vi "GetVehicleOrder.vi"(0 "Input String":string) -> (2 "Lane Offset":dbl, 3 "X":dbl, 4 "Y":dbl, 5 "Yaw":dbl, 14 "Vehicle Id":i32, 15 "Lane String":string, 16 "Is Cruise Control":bool, 17 "Velocity Value":dbl format="%#_13g", 18 "Desired Distance":dbl, 19 "Current Distance":dbl)   [LabVIEW 2013]
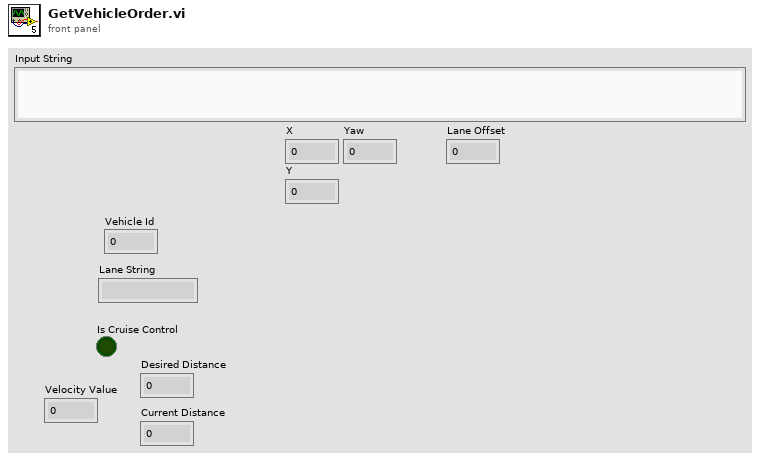
[diagram p1: front panel]
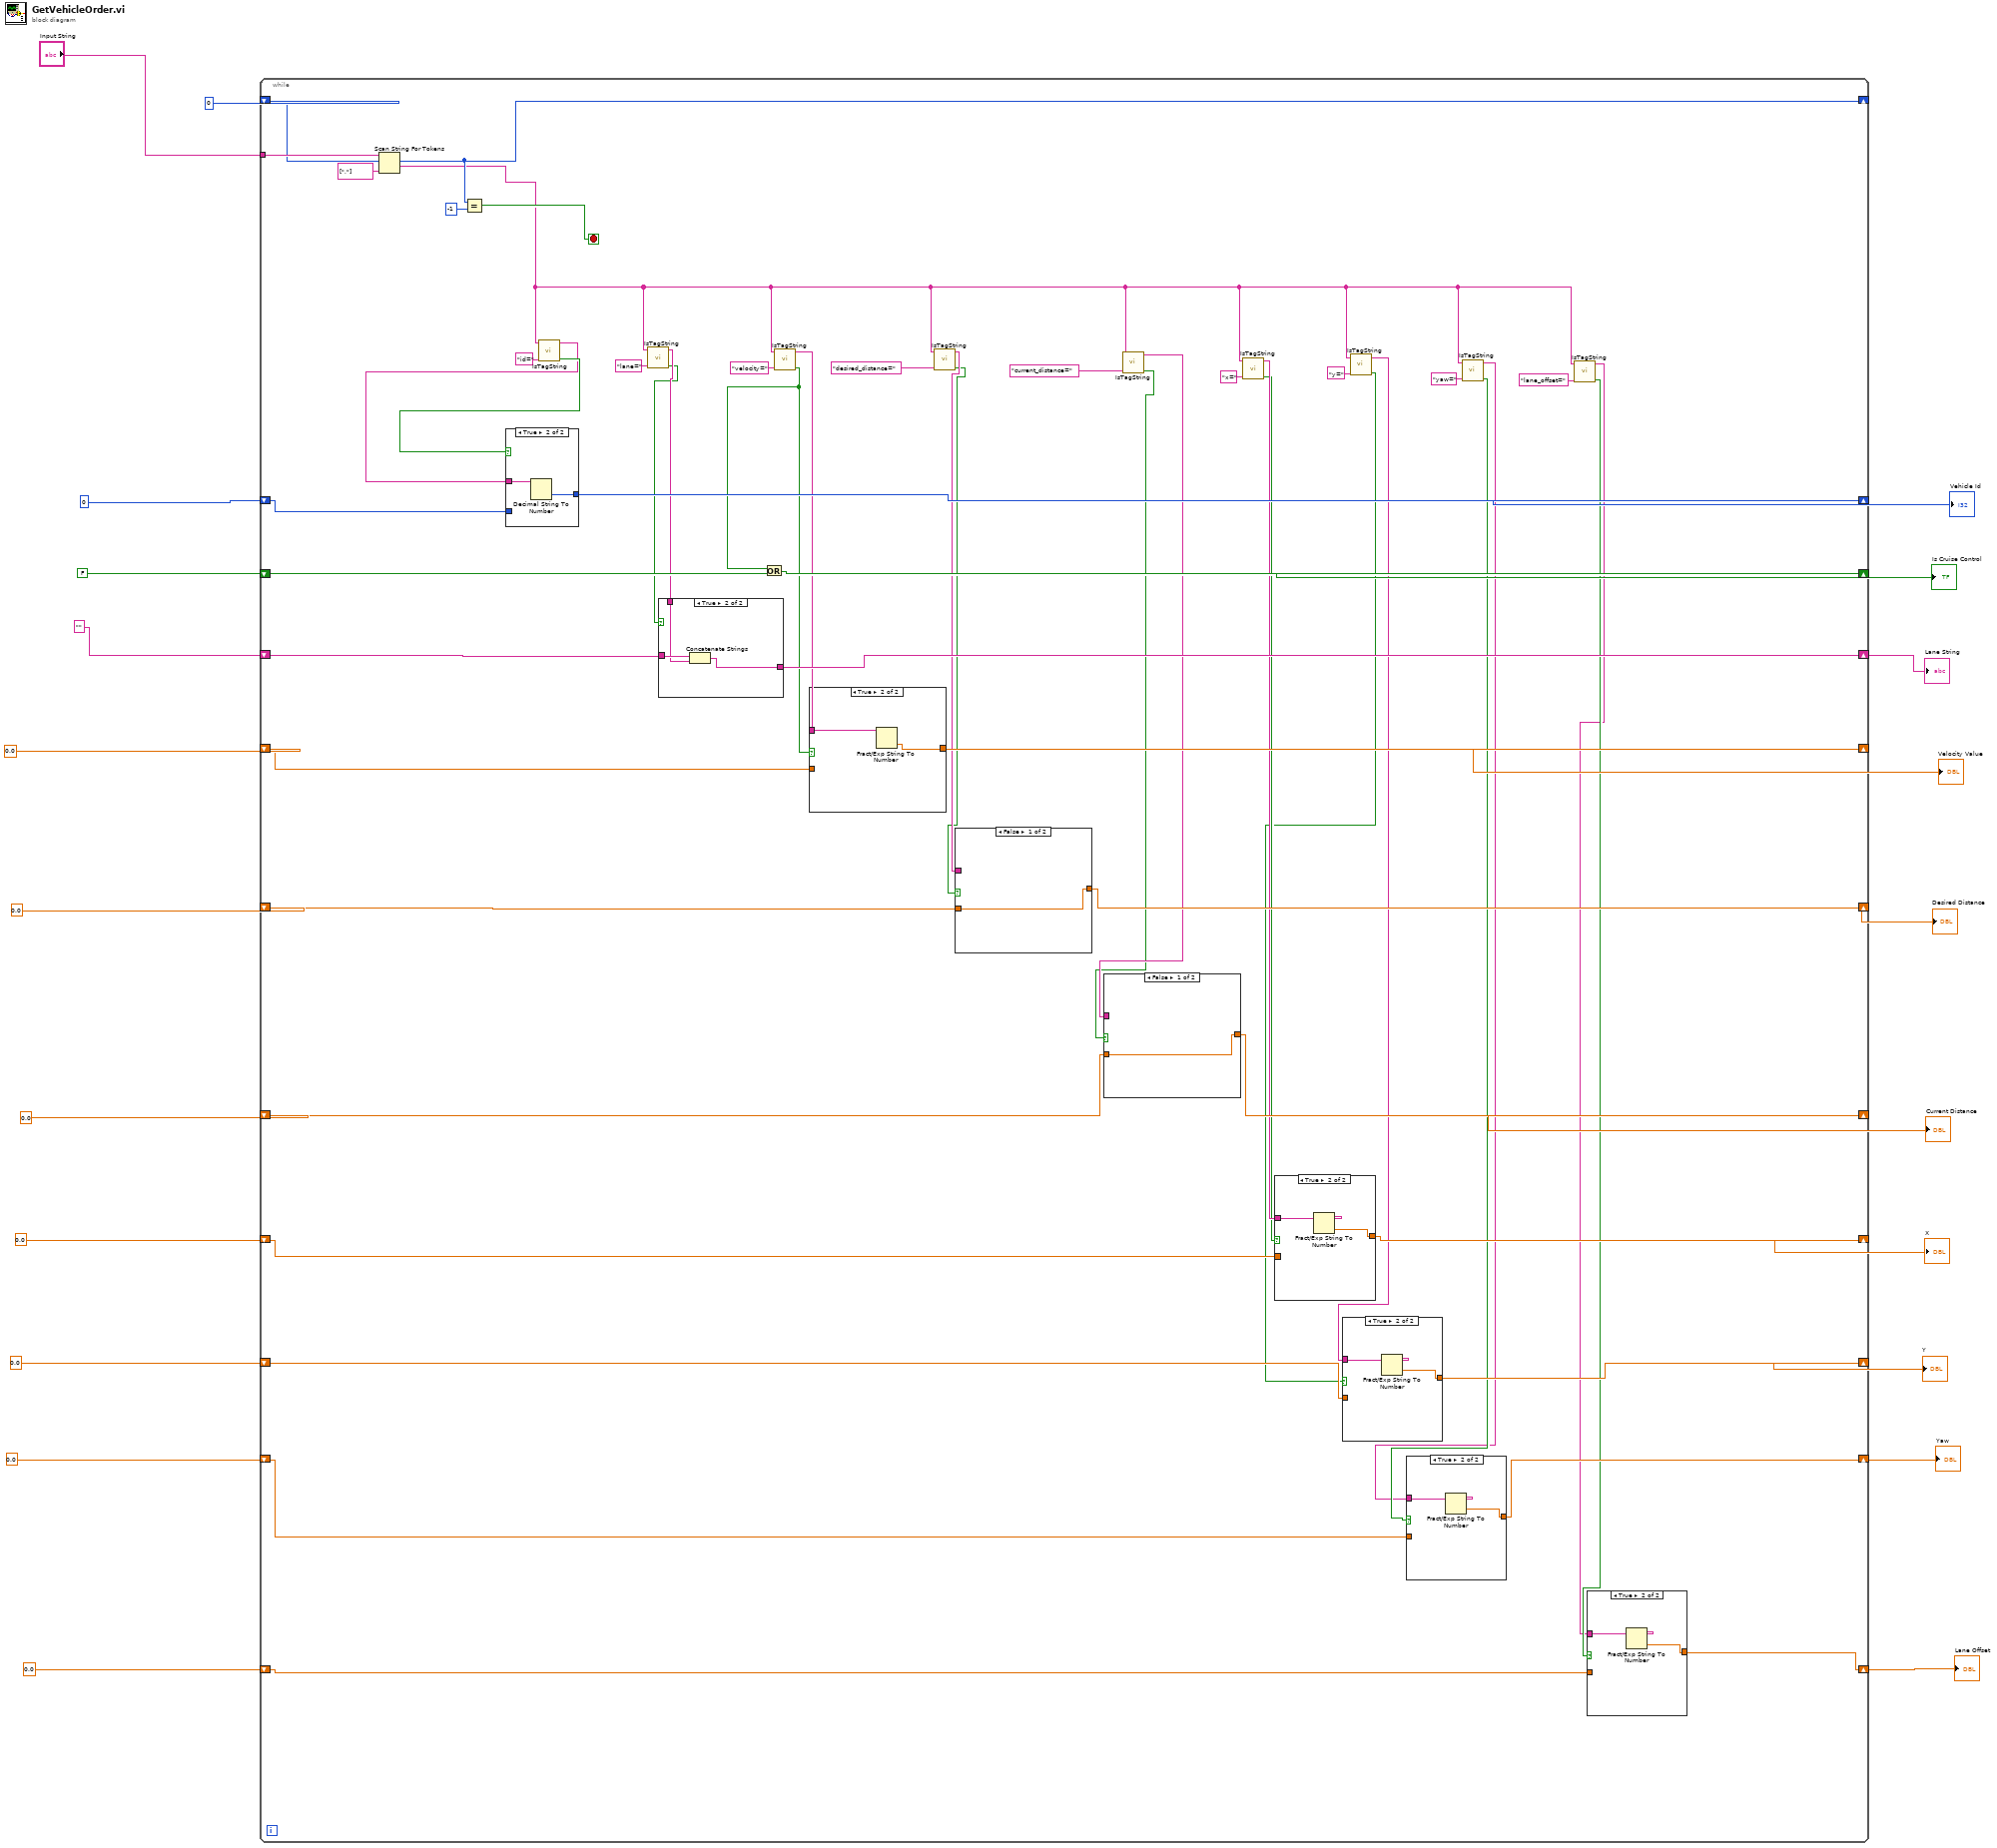
[diagram p0: block diagram]
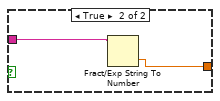
[diagram p6: hidden frame]
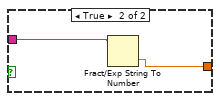
[diagram p7: hidden frame]
diagram:
  n1 = while {
    tunnel: "Input String" -> [w76]
    shift-right: [w49] -> _
    shift-left: 0 -> [w73]
    shift-right: [w66] -> w19
    shift-left: 0 -> [w65]
    shift-right: [w63] -> w17
    shift-left: FALSE -> [w64]
    shift-right: [w60] -> w16
    shift-left: "" -> [w61]
    shift-right: [w58] -> w14
    shift-left: 0.0 -> [w57]
    shift-right: [w55] -> w11
    shift-left: 0.0 -> [w56]
    shift-right: [w54] -> w10
    shift-left: 0.0 -> [w46]
    shift-right: [w37] -> w5
    shift-left: 0.0 -> [w38]
    shift-right: [w36] -> w4
    shift-left: 0.0 -> [w35]
    shift-right: [w33] -> w3
    shift-left: 0.0 -> [w34]
    shift-right: [w28] -> w1
    shift-left: 0.0 -> [w27]
    stop <- w74 stop-if-true
    n2 = Scan String For Tokens(6:string[] [","] ("delimiters (\\s,\\t,\\r,\\n)"), 8:w73, 9:w76) -> (1:w25:string, 2:w49:i32)  [unwired: 3 in, 2 out]
    n3 = Equal?(x=w49, y=-1) -> (x = y?=w74:bool)
    n4 = call "IsTagString.vi"("Input String"=w25, "Tag Desired"="id=") -> ("Value String"=w67:string, "Is Tag String"=w68:bool)  [unwired: 7 in]
    n5 = case shown="True" w68 {
      tunnel: w67 -> [_ w104]
      tunnel: [w102 w103] -> w66
      tunnel: w65 -> [w102 _]
      frame False {
      }
      frame True {
        n6 = Decimal String To Number(string=w104) -> (number=w103:i32)  [unwired: 2 in, 1 out]
      }
    }
    n7 = call "IsTagString.vi"("Input String"=w25, "Tag Desired"="lane=") -> ("Value String"=w62:string, "Is Tag String"=w48:bool)  [unwired: 7 in]
    n8 = case shown="True" w48 {
      tunnel: w61 -> [w98 w101]
      tunnel: w62 -> [_ w100]
      tunnel: [w98 w99] -> w60
      frame False {
      }
      frame True {
        n9 = Concatenate Strings(w101, w100) -> (w99:string)
      }
    }
    n10 = call "IsTagString.vi"("Input String"=w25, "Tag Desired"="velocity=") -> ("Value String"=w59:string, "Is Tag String"=w47:bool)  [unwired: 7 in]
    n11 = Or(x=w47, y=w64) -> (x .or. y?=w63:bool)
    n12 = case shown="True" w47 {
      tunnel: w59 -> [_ w97]
      tunnel: [w95 w96] -> w58
      tunnel: w57 -> [w95 _]
      frame False {
      }
      frame True {
        n13 = Fract/Exp String To Number(string=w97) -> (number=w96:dbl)  [unwired: 3 in, 1 out]
      }
    }
    n14 = call "IsTagString.vi"("Input String"=w25, "Tag Desired"="desired_distance=") -> ("Value String"=w53:string, "Is Tag String"=w52:bool)  [unwired: 7 in]
    n15 = case shown="False" w52 {
      tunnel: w53 -> [_ w94]
      tunnel: [w92 w93] -> w55
      tunnel: w56 -> [w92 _]
      frame False {
      }
      frame True {
        n16 = Fract/Exp String To Number(string=w94) -> (number=w93:dbl)  [unwired: 3 in, 1 out]
      }
    }
    n17 = call "IsTagString.vi"("Input String"=w25, "Tag Desired"="current_distance=") -> ("Value String"=w51:string, "Is Tag String"=w50:bool)  [unwired: 7 in]
    n18 = case shown="False" w50 {
      tunnel: w51 -> [_ w91]
      tunnel: [w89 w90] -> w54
      tunnel: w46 -> [w89 _]
      frame False {
      }
      frame True {
        n19 = Fract/Exp String To Number(string=w91) -> (number=w90:dbl)  [unwired: 3 in, 1 out]
      }
    }
    n20 = call "IsTagString.vi"("Input String"=w25, "Tag Desired"="x=") -> ("Value String"=w40:string, "Is Tag String"=w39:bool)  [unwired: 7 in]
    n21 = case shown="True" w39 {
      tunnel: w40 -> [_ w88]
      tunnel: [w86 w87] -> w37
      tunnel: w38 -> [w86 _]
      frame False {
      }
      frame True {
        n22 = Fract/Exp String To Number(string=w88) -> (number=w87:dbl)  [unwired: 3 in, 1 out]
      }
    }
    n23 = call "IsTagString.vi"("Input String"=w25, "Tag Desired"="y=") -> ("Value String"=w32:string, "Is Tag String"=w31:bool)  [unwired: 7 in]
    n24 = case shown="True" w31 {
      tunnel: w32 -> [_ w85]
      tunnel: [w83 w84] -> w36
      tunnel: w35 -> [w83 _]
      frame False {
      }
      frame True {
        n25 = Fract/Exp String To Number(string=w85) -> (number=w84:dbl)  [unwired: 3 in, 1 out]
      }
    }
    n26 = call "IsTagString.vi"("Input String"=w25, "Tag Desired"="yaw=") -> ("Value String"=w29:string, "Is Tag String"=w30:bool)  [unwired: 7 in]
    n27 = case shown="True" w30 {
      tunnel: w29 -> [_ w82]
      tunnel: [w80 w81] -> w33
      tunnel: w34 -> [w80 _]
      frame False {
      }
      frame True {
        n28 = Fract/Exp String To Number(string=w82) -> (number=w81:dbl)  [unwired: 3 in, 1 out]
      }
    }
    n29 = call "IsTagString.vi"("Input String"=w25, "Tag Desired"="lane_offset=") -> ("Value String"=w23:string, "Is Tag String"=w24:bool)  [unwired: 7 in]
    n30 = case shown="True" w24 {
      tunnel: w23 -> [_ w79]
      tunnel: [w77 w78] -> w28
      tunnel: w27 -> [w77 _]
      frame False {
      }
      frame True {
        n31 = Fract/Exp String To Number(string=w79) -> (number=w78:dbl)  [unwired: 3 in, 1 out]
      }
    }
  }
  "Vehicle Id" <- w19
  "Is Cruise Control" <- w17
  "Lane String" <- w16
  "Velocity Value" <- w14
  "Desired Distance" <- w11
  "Current Distance" <- w10
  "X" <- w5
  "Y" <- w4
  "Yaw" <- w3
  "Lane Offset" <- w1
